vi "Main.vi"(8 "error in (no error)":errorcluster, 11 "ImageStackBase in":refnum<class "Invivo_ImageStack.lvclass">) -> (0 "error out":errorcluster, 3 "component":refnum<class "Invivo_ImageStack.lvclass">)   [LabVIEW 2012, in "Invivo_ImageStack.lvclass"]
doc: "Main VI of the component."
uses:
  Invivo_ImageStack.lvclass
  <vilib>/Distrio/Murmex/Murmex/command_enum.ctl
  Invivo_ImageStack.lvclass/Invivo_ImageStack.ctl
  <vilib>/Distrio/Murmex/InitialiseMessage/InitialiseMessage.lvclass
  <vilib>/Distrio/Murmex/Murmex/data_compression_enum.ctl
  <vilib>/Distrio/Murmex/TerminateMessage/TerminateMessage.lvclass
  <vilib>/Distrio/Murmex/ConfigureMessage/ConfigureMessage.lvclass
  <vilib>/Distrio/Murmex/Murmex/update_cluster.ctl
  <vilib>/Distrio/Murmex/StartMessage/StartMessage.lvclass
  <vilib>/Distrio/Murmex/StopMessage/StopMessage.lvclass
  <vilib>/Distrio/Murmex/Murmex/Set configure at initialise.vi
  <vilib>/Distrio/Murmex/Murmex/Set log reference.vi
  <vilib>/Distrio/Murmex/Murmex/Set VI reference.vi
  <vilib>/Distrio/Murmex/Murmex/Set relay start stop to observers.vi
  <vilib>/Distrio/Murmex/Murmex/Set data compression.vi
  <vilib>/Distrio/Murmex/Murmex/Murmex.lvclass
  <vilib>/Distrio/Murmex/Message/Message.lvclass
panel:
  in  "button:config":bool
  in  "Tab Control":enum32{"User", "Debug", "About"}(tab)
  in  "wait b4 acquisition":dbl[unit]=1.0
  in  "button::direction":bool
  in  "File name":string
  out "Translation speed":dbl[unit]
  in  "button:start":bool
  in  "No. of frames":u16=100
  out "Frame rate":dbl[unit]
  in  "Subfolder levels":string[](array[string])
  in  "Step size":dbl[unit]
  out "log":string
  in  "ID":string="stack"
  in  "button:send command":bool
  in  "Generic command":string
  in  "command":T1
  in  "button:quit":bool
  in  "terminate?":bool=TRUE
  # "ImageStack\n\nImplemented by:\nLudovico Silvestri\nUniversity of Florence, Italy"
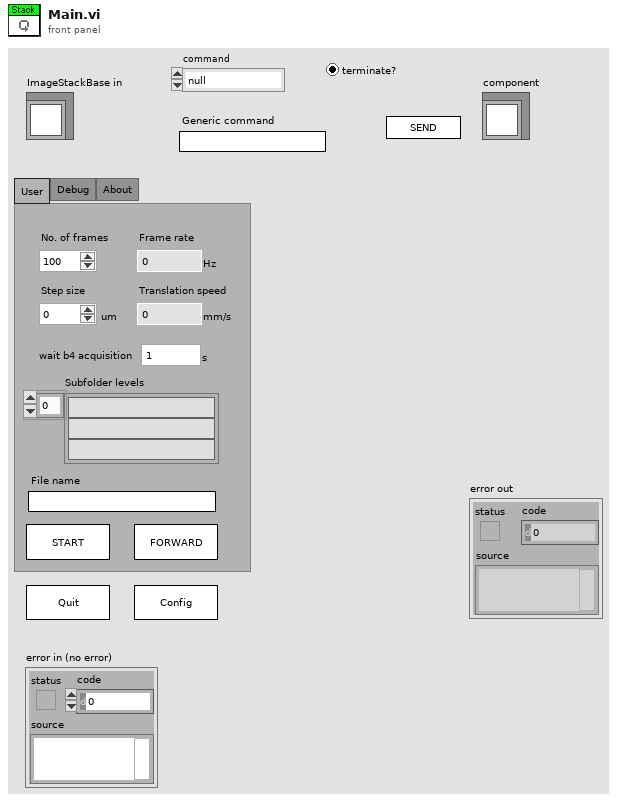
[diagram p1: front panel]
types:
  T1 = typedef "Murmex.lvlib/Murmex.lvclass/command_enum.ctl" = enum16{"null", "initialise", "reset", "terminate", "acknowledge", "update", "inspect", "inform", "proceed", "start", "stop", "fetch", "configure", "generic"}
  T2 = typedef "Murmex.lvlib/Murmex.lvclass/data_compression_enum.ctl" = enum16{"base64", "zip+base64", "byte to string"}
  T3 = typedef "Murmex.lvlib/Murmex.lvclass/update_cluster.ctl" = cluster{"target ID":string, "key chains":string[], "values":variant[]}
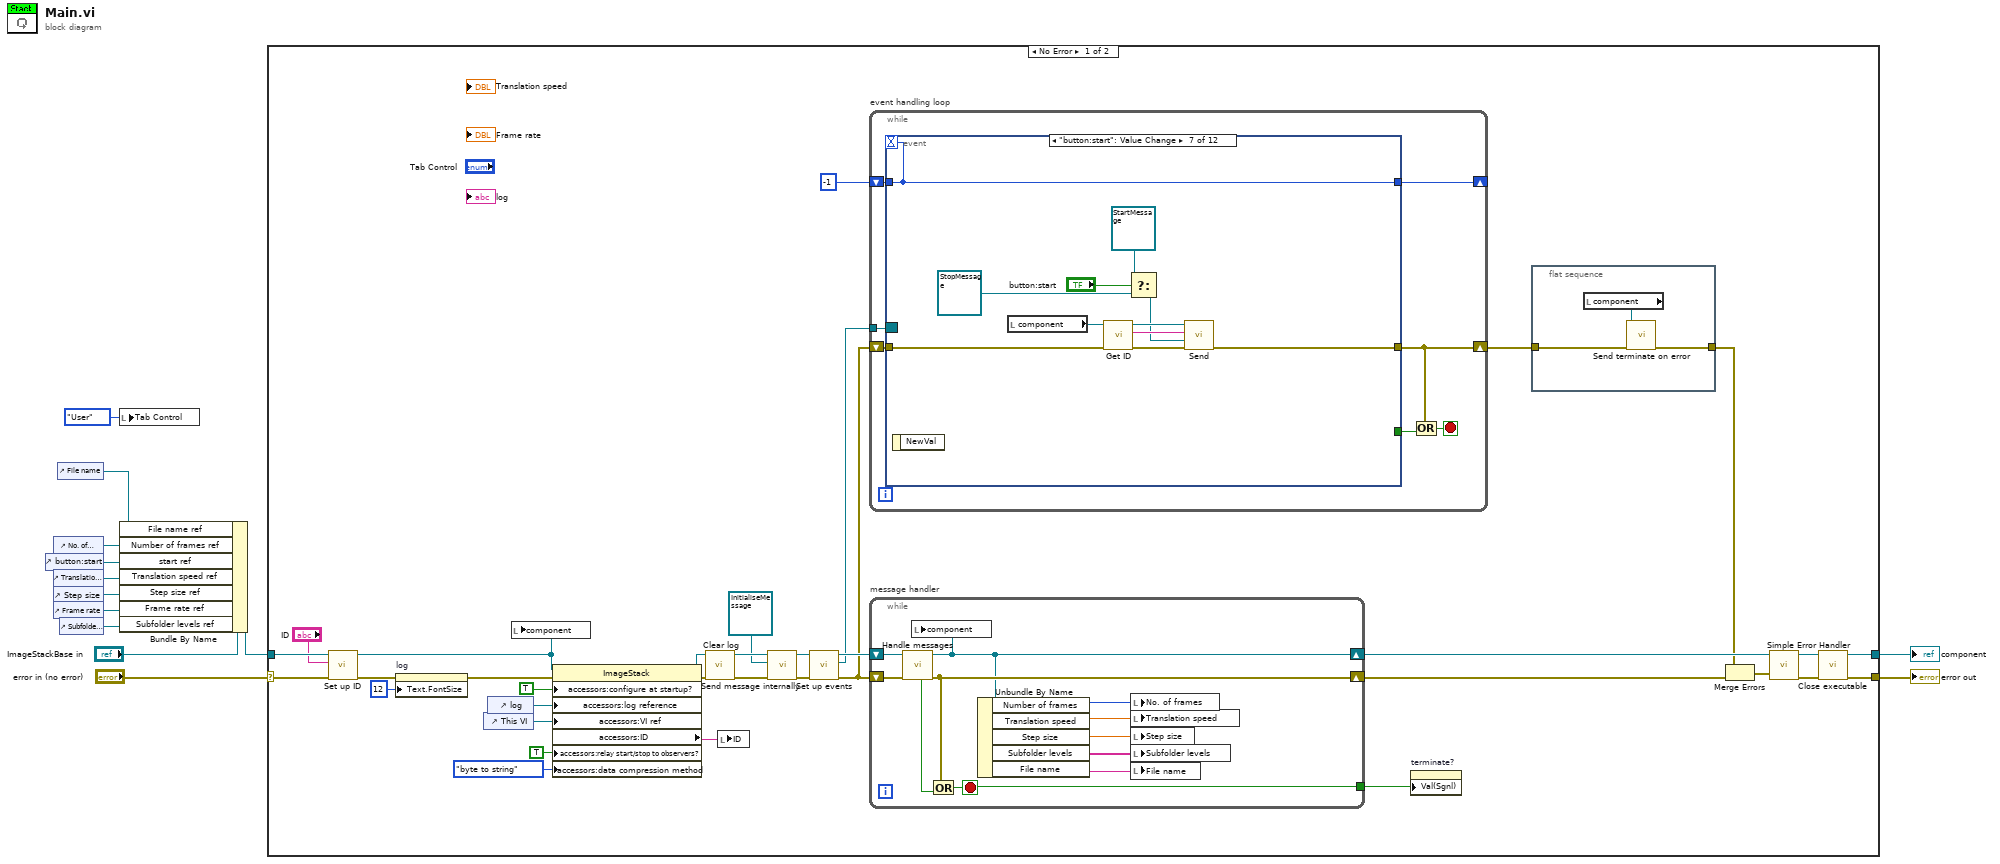
[diagram p0: block diagram]
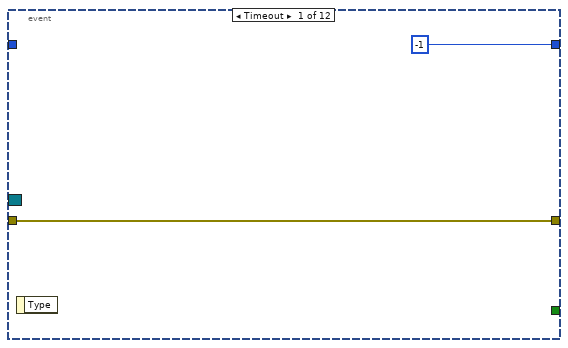
[diagram p2: hidden frame]
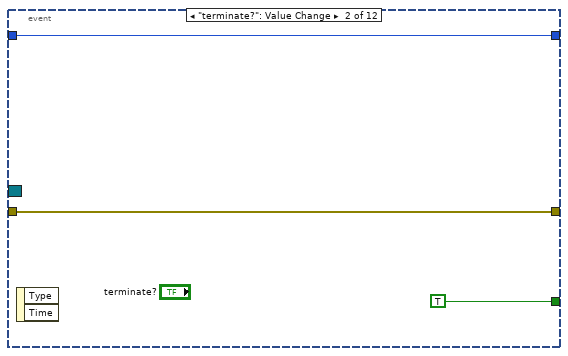
[diagram p3: hidden frame]
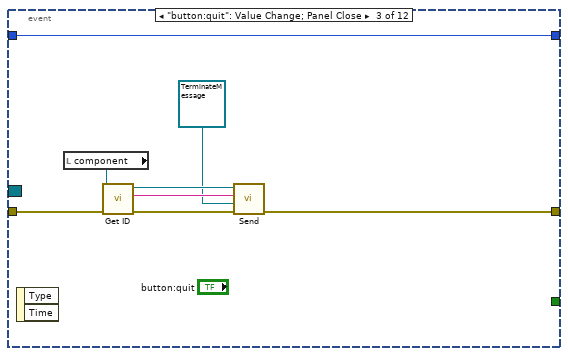
[diagram p4: hidden frame]
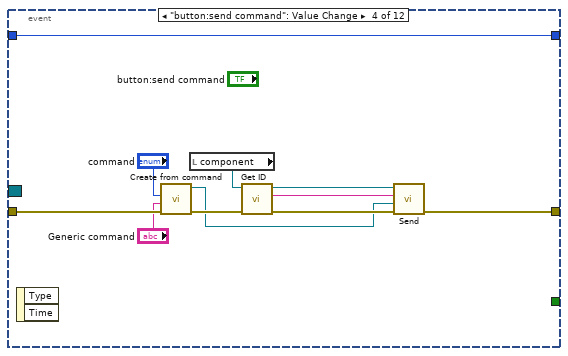
[diagram p5: hidden frame]
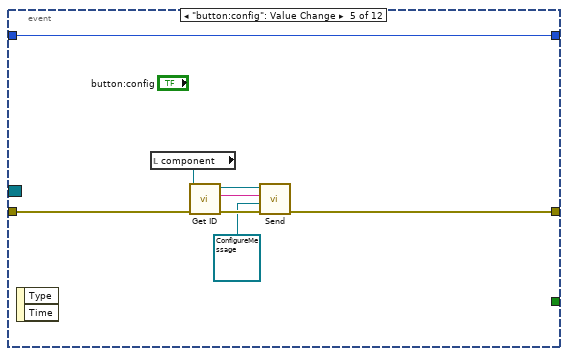
[diagram p6: hidden frame]
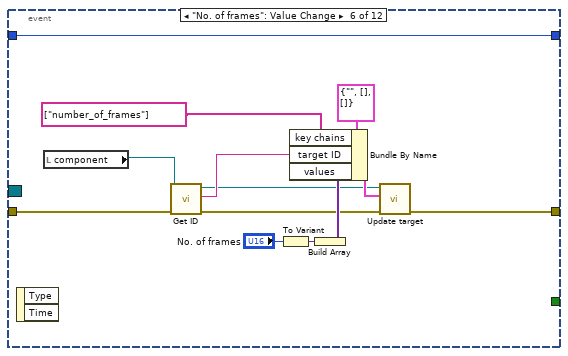
[diagram p7: hidden frame]
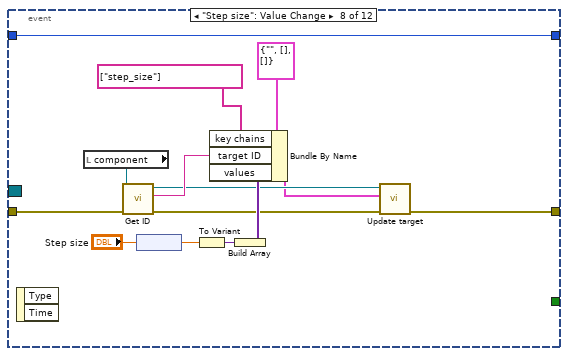
[diagram p8: hidden frame]
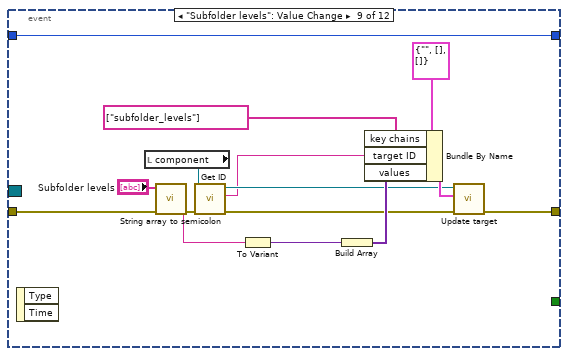
[diagram p9: hidden frame]
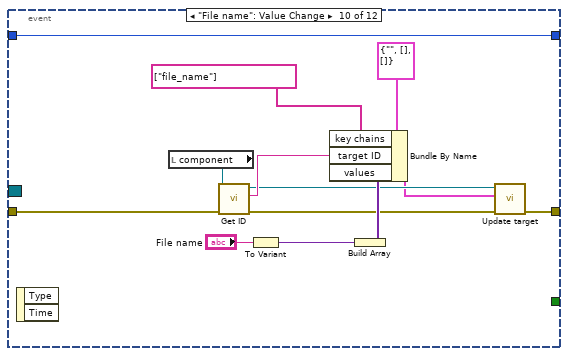
[diagram p10: hidden frame]
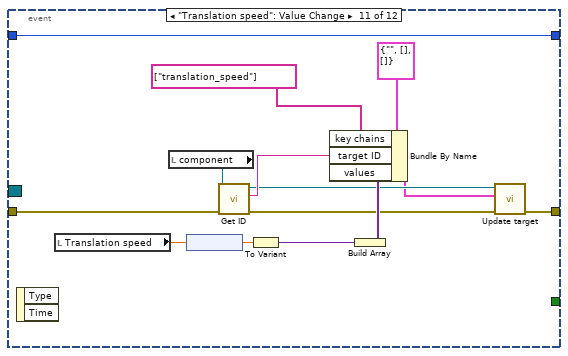
[diagram p11: hidden frame]
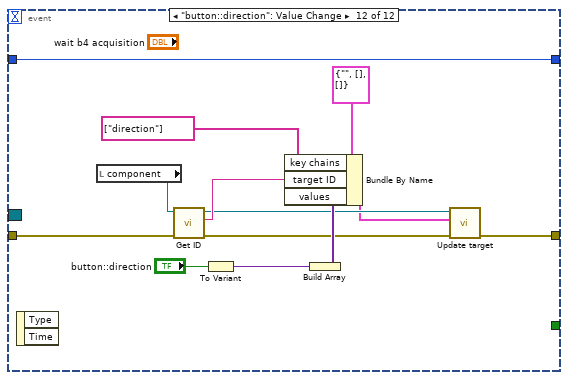
[diagram p12: hidden frame]
diagram:
  n1 = control-ref of="button:start"() -> (w4:refnum<vi>)
  n2 = control-ref of="No. of frames"() -> (w3:refnum<vi>)
  n3 = control-ref of="Translation speed"() -> (w5:refnum<vi>)
  n4 = control-ref of="Step size"() -> (w6:refnum<vi>)
  n5 = control-ref of="Frame rate"() -> (w7:refnum<vi>)
  n6 = control-ref of="File name"() -> (w1:refnum<vi>)
  n7 = control-ref of="Subfolder levels"() -> (w8:refnum<vi>)
  n8 = local write "Tab Control"(enum32{"User", "Debug", "About"}."User" ("Tab Control")) -> ()
  n9 = Bundle By Name(cluster="ImageStackBase in", "File name ref"=w1, "Number of frames ref"=w3, "start ref"=w4, "Translation speed ref"=w5, "Step size ref"=w6, "Frame rate ref"=w7, "Subfolder levels ref"=w8) -> (w9:refnum<class "Invivo_ImageStack.lvclass">)
  n10 = case shown="No Error" "error in (no error)" {
    selector: "error in (no error)" -> [w38 w193]
    tunnel: w9 -> [w37 w194]
    tunnel: [w16 w194] -> w11
    tunnel: [w17 w193] -> w10
    frame No Error {
      n11 = call <vilib>:"Set up ID.vi"("error in (no error)"=w38, "component ID"="ID", "MurmexBase in"=w37) -> ("error out"=w26:errorcluster, "MurmexBase out"=w34:refnum<class "Invivo_ImageStack.lvclass">)  [unwired: 6 in, 1 out]
      n12 = property on="log" class="Str"(error in=w26, "Text.FontSize"=u32 12 ("Text.Font:Size")) -> (error out=w25:errorcluster)  [unwired: 1 in, 1 out]
      n13 = control-ref of="This VI"() -> (w44:refnum<vi>)
      n14 = control-ref of="log"() -> (w45:refnum<vi>)
      n15 = local write "component"(w34) -> ()
      n16 = property class="ImageStack"(reference=w34, error in=w25, "accessors:configure at startup?"=TRUE ("configure at startup?"), "accessors:log reference"=w45, "accessors:VI ref"=w44, "accessors:relay start/stop to observers?"=TRUE ("relay start/stop to observers?"), "accessors:data compression method"=data_compression_enum."byte to string" ("data compression method")) -> (reference out=w43:refnum<class "Invivo_ImageStack.lvclass">, error out=w42:errorcluster, "accessors:ID"=w35:string)
      n17 = call <vilib>:"Clear log.vi"("error in (no error)"=w42, "MurmexBase in"=w43) -> ("error out"=w41:errorcluster, "MurmexBase out"=w40:refnum<class "Invivo_ImageStack.lvclass">)  [unwired: 8 in]
      n18 = local write "ID"(w35) -> ()
      n19 = call <vilib>:"Send message internally.vi"("error in (no error)"=w41, "Message"=refnum<class "InitialiseMessage.lvclass"> refnum ("Murmex.lvlib:InitialiseMessage"), "Murmex in"=w40) -> ("error out"=w33:errorcluster, "Murmex out"=w32:refnum<class "Invivo_ImageStack.lvclass">)  [unwired: 7 in]
      n20 = call <vilib>:"Set up events.vi"("error in (no error)"=w33, "MurmexBase in"=w32) -> ("error out"=w29:errorcluster, "Event Registration Refnum"=w28:refnum<event-registration>, "MurmexBase out"=w31:refnum<class "Invivo_ImageStack.lvclass">)  [unwired: 7 in]
      n21 = while "event handling loop" {
        shift-right: [w55] -> _
        shift-left: -1 -> [w56]
        shift-right: [w51] -> w19
        shift-left: w29 -> [w54]
        tunnel: w28 -> [w53]
        stop <- w52 stop-if-true
        n22 = event shown="[6] \"button:start\": Value Change" {
          selector: w53 -> [_ _ _ _ _ _ _ _ _ _ _ _]
          dyn-events: _ -> [_ _ _ _ _ _ _ _ _ _ _ _]
          timeout: w56 -> [_ _ _ _ _ _ _ _ _ _ _ _]
          tunnel: w56 -> [_ w59 w62 w70 w81 w97 w102 w114 w136 w144 w158 w169]
          tunnel: [-1 w59 w62 w70 w81 w97 w102 w114 w136 w144 w158 w169] -> w55
          tunnel: [w57 w61 w65 w75 w86 w98 w107 w118 w137 w147 w161 w171] -> w51
          tunnel: w54 -> [w57 w61 w69 w80 w88 w100 w108 w124 w135 w143 w157 w173]
          tunnel: [_ TRUE _ _ _ _ _ _ _ _ _ _] -> w50
          event Timeout {
            n23 = event-data() -> ()  [unwired: 1 in, 1 out]
          }
          event "terminate?": Value Change {
            n24 = event-data() -> ()  [unwired: 1 in, 2 out]
          }
          event "button:quit": Value Change; Panel Close {
            n25 = event-data() -> ()  [unwired: 1 in, 2 out]
            n26 = local read "component"() -> (w68:refnum<class "Invivo_ImageStack.lvclass">)
            n27 = call <vilib>:"Get ID.vi"("error in (no error)"=w69, "Murmex in"=w68) -> ("error out"=w66:errorcluster, "component id"=w64:string, "Murmex out"=w67:refnum<class "Invivo_ImageStack.lvclass">)  [unwired: 7 in]
            n28 = call <vilib>:"Send.vi"("error in (no error)"=w66, "Message"=refnum<class "TerminateMessage.lvclass"> refnum ("Murmex.lvlib:TerminateMessage"), "recipient"=w64, "Murmex in"=w67) -> ("error out"=w65:errorcluster)  [unwired: 6 in, 1 out]
          }
          event "button:send command": Value Change {
            n29 = event-data() -> ()  [unwired: 1 in, 2 out]
            n30 = call <vilib>:"Create from command.vi"("error in (no error)"=w80, "generic command"="Generic command", "command"="command") -> ("error out"=w77:errorcluster, "Message out"=w74:refnum<class "Message.lvclass">)  [unwired: 7 in]
            n31 = local read "component"() -> (w73:refnum<class "Invivo_ImageStack.lvclass">)
            n32 = call <vilib>:"Get ID.vi"("error in (no error)"=w77, "Murmex in"=w73) -> ("error out"=w76:errorcluster, "component id"=w71:string, "Murmex out"=w72:refnum<class "Invivo_ImageStack.lvclass">)  [unwired: 7 in]
            n33 = call <vilib>:"Send.vi"("error in (no error)"=w76, "Message"=w74, "recipient"=w71, "Murmex in"=w72) -> ("error out"=w75:errorcluster)  [unwired: 6 in, 1 out]
          }
          event "button:config": Value Change {
            n34 = event-data() -> ()  [unwired: 1 in, 2 out]
            n35 = local read "component"() -> (w82:refnum<class "Invivo_ImageStack.lvclass">)
            n36 = call <vilib>:"Get ID.vi"("error in (no error)"=w88, "Murmex in"=w82) -> ("error out"=w87:errorcluster, "component id"=w84:string, "Murmex out"=w85:refnum<class "Invivo_ImageStack.lvclass">)  [unwired: 7 in]
            n37 = call <vilib>:"Send.vi"("error in (no error)"=w87, "Message"=refnum<class "ConfigureMessage.lvclass"> refnum ("Murmex.lvlib:ConfigureMessage"), "recipient"=w84, "Murmex in"=w85) -> ("error out"=w86:errorcluster)  [unwired: 6 in, 1 out]
          }
          event "No. of frames": Value Change {
            n38 = event-data() -> ()  [unwired: 1 in, 2 out]
            n39 = local read "component"() -> (w99:refnum<class "Invivo_ImageStack.lvclass">)
            n40 = call <vilib>:"Get ID.vi"("error in (no error)"=w100, "Murmex in"=w99) -> ("error out"=w89:errorcluster, "component id"=w91:string, "Murmex out"=w90:refnum<class "Invivo_ImageStack.lvclass">)  [unwired: 7 in]
            n41 = To Variant(anything="No. of frames") -> (Variant=w94:variant)
            n42 = Build Array(w94) -> (w93:variant[])
            n43 = Bundle By Name(cluster=T3 {"target ID"="", "key chains"=[], "values"=[]} ("update cluster"), "key chains"=string[] ["number_of_frames"], "target ID"=w91, "values"=w93) -> (w92:T3)
            n44 = call <vilib>:"Update target.vi"("error in (no error)"=w89, "update cluster"=w92, "MurmexBase in"=w90) -> ("error out"=w98:errorcluster)  [unwired: 7 in, 1 out]
          }
          event "button:start": Value Change {
            n45 = event-data() -> ()  [unwired: 1 in, 1 out]
            n46 = local read "component"() -> (w109:refnum<class "Invivo_ImageStack.lvclass">)
            n47 = call <vilib>:"Get ID.vi"("error in (no error)"=w108, "Murmex in"=w109) -> ("error out"=w112:errorcluster, "component id"=w110:string, "Murmex out"=w111:refnum<class "Invivo_ImageStack.lvclass">)  [unwired: 7 in]
            n48 = Select(t=refnum<class "StartMessage.lvclass"> refnum ("Message in"), s="button:start", f=refnum<class "StopMessage.lvclass"> refnum ("Distrio Murmex 1.0:StopMessage")) -> (s? t:f=w104:refnum<class "Message.lvclass">)
            n49 = call <vilib>:"Send.vi"("error in (no error)"=w112, "Message"=w104, "recipient"=w110, "Murmex in"=w111) -> ("error out"=w107:errorcluster)  [unwired: 6 in, 1 out]
          }
          event "Step size": Value Change {
            n50 = event-data() -> ()  [unwired: 1 in, 2 out]
            n51 = local read "component"() -> (w120:refnum<class "Invivo_ImageStack.lvclass">)
            n52 = call <vilib>:"Get ID.vi"("error in (no error)"=w124, "Murmex in"=w120) -> ("error out"=w119:errorcluster, "component id"=w123:string, "Murmex out"=w117:refnum<class "Invivo_ImageStack.lvclass">)  [unwired: 7 in]
            n53 = node("Step size") -> (w113:dbl)
            n54 = To Variant(anything=w113) -> (Variant=w122:variant)
            n55 = Build Array(w122) -> (w121:variant[])
            n56 = Bundle By Name(cluster=T3 {"target ID"="", "key chains"=[], "values"=[]} ("update cluster"), "key chains"=string[] ["step_size"], "target ID"=w123, "values"=w121) -> (w116:T3)
            n57 = call <vilib>:"Update target.vi"("error in (no error)"=w119, "update cluster"=w116, "MurmexBase in"=w117) -> ("error out"=w118:errorcluster)  [unwired: 7 in, 1 out]
          }
          event "Subfolder levels": Value Change {
            n58 = event-data() -> ()  [unwired: 1 in, 2 out]
            n59 = local read "component"() -> (w138:refnum<class "Invivo_ImageStack.lvclass">)
            n60 = call "String array to semicolon.vi"("error in"=w135, "String array"="Subfolder levels") -> ("error out"=w134:errorcluster, "Semicolon string"=w132:string)  [unwired: 8 in]
            n61 = call <vilib>:"Get ID.vi"("error in (no error)"=w134, "Murmex in"=w138) -> ("error out"=w128:errorcluster, "component id"=w127:string, "Murmex out"=w129:refnum<class "Invivo_ImageStack.lvclass">)  [unwired: 7 in]
            n62 = To Variant(anything=w132) -> (Variant=w139:variant)
            n63 = Build Array(w139) -> (w131:variant[])
            n64 = Bundle By Name(cluster=T3 {"target ID"="", "key chains"=[], "values"=[]} ("update cluster"), "key chains"=string[] ["subfolder_levels"], "target ID"=w127, "values"=w131) -> (w130:T3)
            n65 = call <vilib>:"Update target.vi"("error in (no error)"=w128, "update cluster"=w130, "MurmexBase in"=w129) -> ("error out"=w137:errorcluster)  [unwired: 7 in, 1 out]
          }
          event "File name": Value Change {
            n66 = event-data() -> ()  [unwired: 1 in, 2 out]
            n67 = local read "component"() -> (w149:refnum<class "Invivo_ImageStack.lvclass">)
            n68 = call <vilib>:"Get ID.vi"("error in (no error)"=w143, "Murmex in"=w149) -> ("error out"=w148:errorcluster, "component id"=w152:string, "Murmex out"=w146:refnum<class "Invivo_ImageStack.lvclass">)  [unwired: 7 in]
            n69 = To Variant(anything="File name") -> (Variant=w151:variant)
            n70 = Build Array(w151) -> (w150:variant[])
            n71 = Bundle By Name(cluster=T3 {"target ID"="", "key chains"=[], "values"=[]} ("update cluster"), "key chains"=string[] ["file_name"], "target ID"=w152, "values"=w150) -> (w145:T3)
            n72 = call <vilib>:"Update target.vi"("error in (no error)"=w148, "update cluster"=w145, "MurmexBase in"=w146) -> ("error out"=w147:errorcluster)  [unwired: 7 in, 1 out]
          }
          event "Translation speed": Value Change {
            n73 = event-data() -> ()  [unwired: 1 in, 2 out]
            n74 = local read "Translation speed"() -> (w156:dbl[unit])
            n75 = local read "component"() -> (w163:refnum<class "Invivo_ImageStack.lvclass">)
            n76 = node(w156) -> (w155:dbl)
            n77 = call <vilib>:"Get ID.vi"("error in (no error)"=w157, "Murmex in"=w163) -> ("error out"=w162:errorcluster, "component id"=w166:string, "Murmex out"=w160:refnum<class "Invivo_ImageStack.lvclass">)  [unwired: 7 in]
            n78 = To Variant(anything=w155) -> (Variant=w165:variant)
            n79 = Build Array(w165) -> (w164:variant[])
            n80 = Bundle By Name(cluster=T3 {"target ID"="", "key chains"=[], "values"=[]} ("update cluster"), "key chains"=string[] ["translation_speed"], "target ID"=w166, "values"=w164) -> (w159:T3)
            n81 = call <vilib>:"Update target.vi"("error in (no error)"=w162, "update cluster"=w159, "MurmexBase in"=w160) -> ("error out"=w161:errorcluster)  [unwired: 7 in, 1 out]
          }
          event "button::direction": Value Change {
            n82 = event-data() -> ()  [unwired: 1 in, 2 out]
            n83 = local read "component"() -> (w172:refnum<class "Invivo_ImageStack.lvclass">)
            n84 = call <vilib>:"Get ID.vi"("error in (no error)"=w173, "Murmex in"=w172) -> ("error out"=w177:errorcluster, "component id"=w180:string, "Murmex out"=w176:refnum<class "Invivo_ImageStack.lvclass">)  [unwired: 7 in]
            n85 = To Variant(anything="button::direction") -> (Variant=w179:variant)
            n86 = Build Array(w179) -> (w178:variant[])
            n87 = Bundle By Name(cluster=T3 {"target ID"="", "key chains"=[], "values"=[]} ("update cluster"), "key chains"=string[] ["direction"], "target ID"=w180, "values"=w178) -> (w175:T3)
            n88 = call <vilib>:"Update target.vi"("error in (no error)"=w177, "update cluster"=w175, "MurmexBase in"=w176) -> ("error out"=w171:errorcluster)  [unwired: 7 in, 1 out]
          }
        }
        n89 = Or(x=w51, y=w50) -> (x .or. y?=w52:bool)
      }
      n90 = while "message handler" {
        shift-right: [w187] -> w15
        shift-left: w31 -> [w192]
        shift-right: [w190] -> w18
        shift-left: w29 -> [w191]
        tunnel: [w188] -> w27
        stop <- w188 stop-if-true
        n91 = call <vilib>:"Handle messages.vi"("error in (no error)"=w191, "Murmex in"=w192) -> ("error out"=w190:errorcluster, "Murmex out"=w187:refnum<class "Invivo_ImageStack.lvclass">, "terminated?"=w189:bool)  [unwired: 7 in]
        n92 = local write "component"(w187) -> ()
        n93 = Or(x=w190, y=w189) -> (x .or. y?=w188:bool)
        n94 = Unbundle By Name(w187) -> ("Number of frames"=w185:u16, "Translation speed"=w186:dbl[unit], "Step size"=w184:dbl[unit], "Subfolder levels"=w183:string[], "File name"=w182:string)
        n95 = local write "No. of frames"(w185) -> ()
        n96 = local write "Translation speed"(w186) -> ()
        n97 = local write "Step size"(w184) -> ()
        n98 = local write "Subfolder levels"(w183) -> ()
        n99 = local write "File name"(w182) -> ()
      }
      n100 = property on="terminate?" class="Bool (strict)"("Val(Sgnl)"=w27) -> ()  [unwired: 2 in, 2 out]
      n101 = flat-sequence {
        tunnel: w19 -> [w49]
        tunnel: [w47] -> w14
        frame #0 {
          n102 = local read "component"() -> (w48:refnum<class "Invivo_ImageStack.lvclass">)
          n103 = call <vilib>:"Send terminate on error.vi"("error in (no error)"=w49, "Murmex in"=w48) -> ("error out"=w47:errorcluster)  [unwired: 8 in, 1 out]
        }
      }
      n104 = Merge Errors(w14, w18) -> (w20:errorcluster)
      n105 = call <vilib>:"Simple Error Handler.vi"("error in (no error)"=w20) -> ("error out"=w21:errorcluster)  [unwired: 4 in, 4 out]
      n106 = call <vilib>:"Close executable.vi"("error in (no error)"=w21, "MurmexBase in"=w15) -> ("error out"=w17:errorcluster, "MurmexBase out"=w16:refnum<class "Invivo_ImageStack.lvclass">)  [unwired: 8 in]
    }
    frame Error {
    }
  }
  "error out" <- w10
  "component" <- w11
